vi "Write Manipulator Control.vi"(8 "error in (no error)":errorcluster, 10 "Manipulator Control":T1, 11 "Supervisor in":refnum<class "Supervisor.lvclass">) -> (0 "error out":errorcluster, 3 "Supervisor out":refnum<class "Supervisor.lvclass">)   [LabVIEW 2014, in "Supervisor.lvclass"]
uses:
  Supervisor.lvclass
  Supervisor.lvclass/Supervisor.ctl
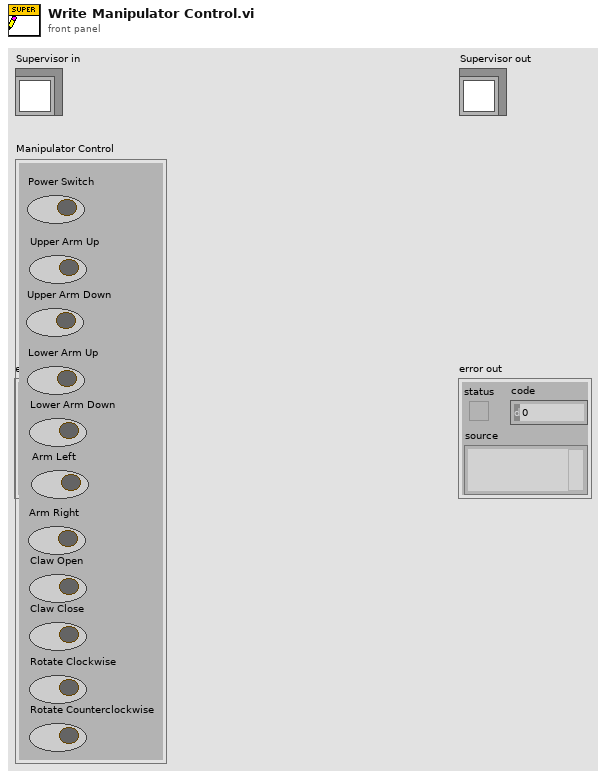
[diagram p1: front panel]
types:
  T1 = cluster{"Power Switch":bool, "Upper Arm Up":bool, "Upper Arm Down":bool, "Lower Arm Up":bool, "Lower Arm Down":bool, "Arm Left":bool, "Arm Right":bool, "Claw Open":bool, "Claw Close":bool, "Rotate Clockwise":bool, "Rotate Counterclockwise":bool}
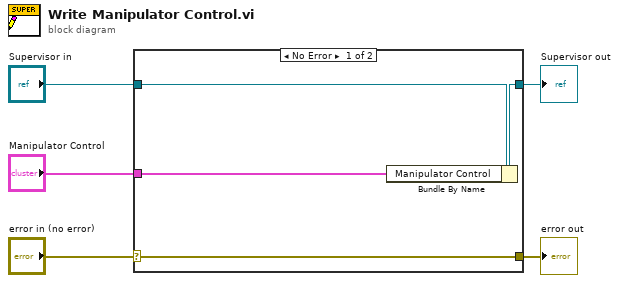
[diagram p0: block diagram]
diagram:
  n1 = case shown="No Error" "error in (no error)" {
    selector: "error in (no error)" -> [w9 w10]
    tunnel: [w9 w10] -> w4
    tunnel: [w7 w11] -> w2
    tunnel: "Supervisor in" -> [w8 w11]
    tunnel: "Manipulator Control" -> [w6 _]
    frame No Error {
      n2 = Bundle By Name(cluster=w8, "Manipulator Control"=w6) -> (w7:refnum<class "Supervisor.lvclass">)
    }
    frame Error {
    }
  }
  "error out" <- w4
  "Supervisor out" <- w2
